vi "micIndividualTest.vi"() -> ()   [LabVIEW 2017]
uses:
  <vilib>/express/express analysis/Spectral/Block/exnSpectralBlock spectral measurements RMS poly.vi
  <vilib>/express/express analysis/Spectral/Block/exnSpectralBlock spectral measurements RMS DDT.vi
  <vilib>/express/express analysis/Spectral/XNode/ExpressSpectralMeasurementsBlockNode.xnode
panel:
  in  "Low pass filter":bool
  in  "Cut-Off Freq":dbl=800.0 caption="Lower Cut-Off"
  in  "Sampling Rate":dbl=25600.0
  in  "Tab Control":T1(tab)=enum."1-4"
  in  "Channel":u16(ring) items=["0", "1", "2", "3", "4", "5", "6", "7", "8", "9", "10", "11", "12", "13", "14", "15", "16"]
  out "Selected mic":dynamicdata(graph) caption="mic_4"
  out "fft selected mic":dynamicdata(graph)
  out "mic_3":dynamicdata(graph)
  out "fft_mic_3":dynamicdata(graph)
  out "fft_mic_4":dynamicdata(graph)
  out "mic_4":dynamicdata(graph)
  out "mic_1":dynamicdata(graph)
  out "fft_mic_1":dynamicdata(graph)
  out "fft_mic_2":dynamicdata(graph)
  out "mic_2":dynamicdata(graph)
  out "mic_6":dynamicdata(graph) caption="mic_2"
  out "fft_mic_6":dynamicdata(graph)
  out "fft_mic_5":dynamicdata(graph)
  out "mic_5":dynamicdata(graph) caption="mic_1"
  out "mic_8":dynamicdata(graph) caption="mic_4"
  out "fft_mic_8":dynamicdata(graph)
  out "fft_mic_7":dynamicdata(graph)
  out "mic_7":dynamicdata(graph) caption="mic_3"
  out "mic_11":dynamicdata(graph) caption="mic_3"
  out "fft_mic_11":dynamicdata(graph)
  out "fft_mic_12":dynamicdata(graph)
  out "mic_12":dynamicdata(graph) caption="mic_4"
  out "mic_9":dynamicdata(graph) caption="mic_1"
  out "fft_mic_9":dynamicdata(graph)
  out "fft_mic_10":dynamicdata(graph)
  out "mic_10":dynamicdata(graph) caption="mic_2"
  out "mic_14":dynamicdata(graph) caption="mic_2"
  out "fft_mic_14":dynamicdata(graph)
  out "fft_mic_13":dynamicdata(graph)
  out "mic_13":dynamicdata(graph) caption="mic_1"
  out "mic_16":dynamicdata(graph) caption="mic_4"
  out "fft_mic_16":dynamicdata(graph)
  out "fft_mic_15":dynamicdata(graph)
  out "mic_15":dynamicdata(graph) caption="mic_3"
  in  "stop (F)":bool caption="Stop (F)"
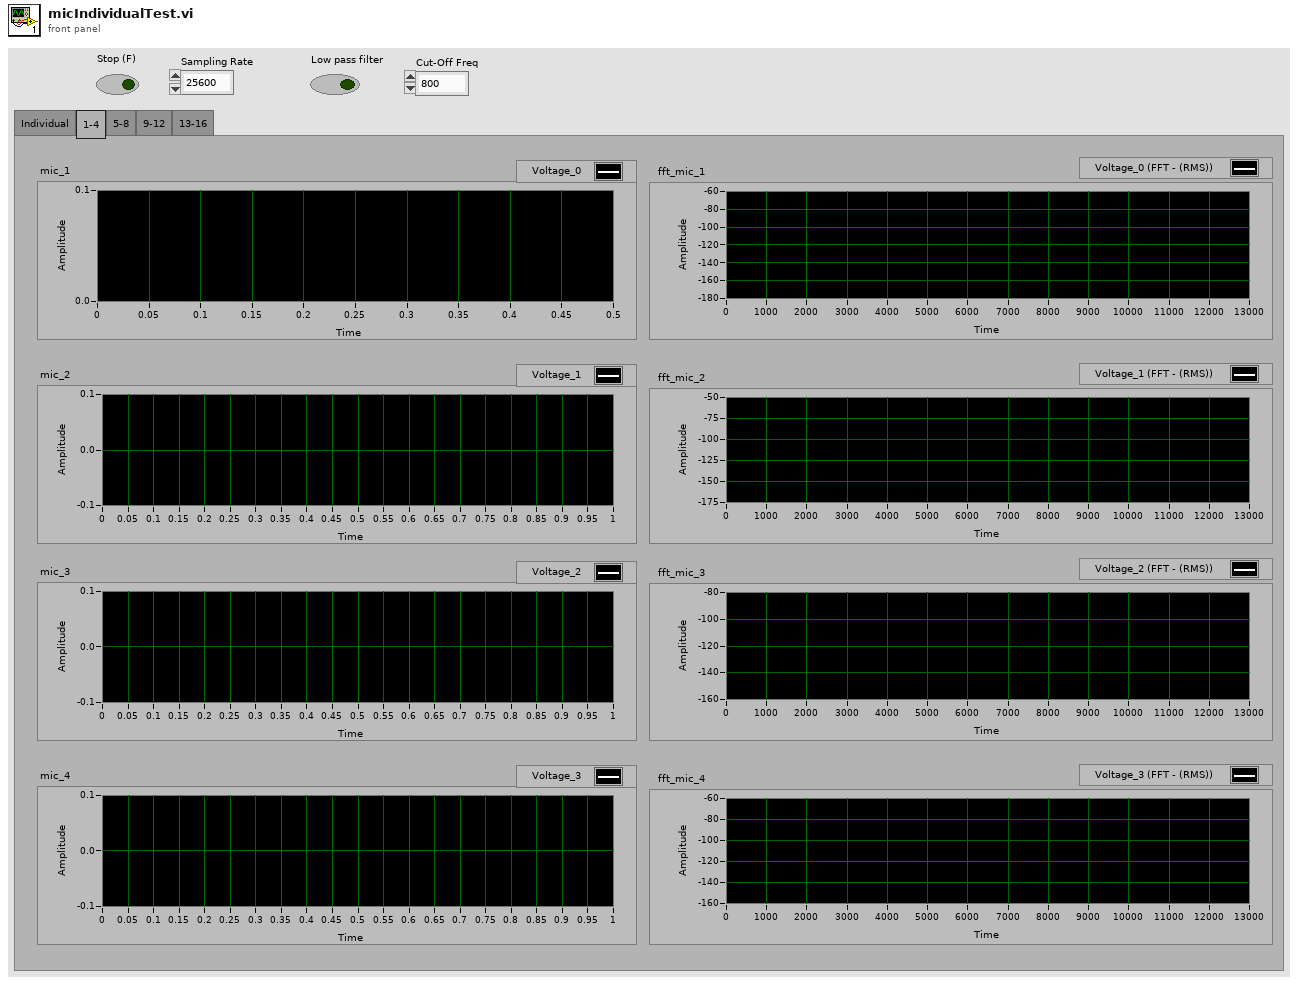
[diagram p1: front panel]
types:
  T1 = enum32{"Individual", "1-4", "5-8", "9-12", "13-16"}
  T2 = cluster{"averaging mode":u16, "weighting mode":u16, "number of averages":u32}
  T3 = cluster{"dB On (F)":bool, "unwrap phase (F)":bool, "convert to degree (F)":bool}
  T4 = enum8{"Enabled", "Disabled", "Disabled and Grayed Out"}
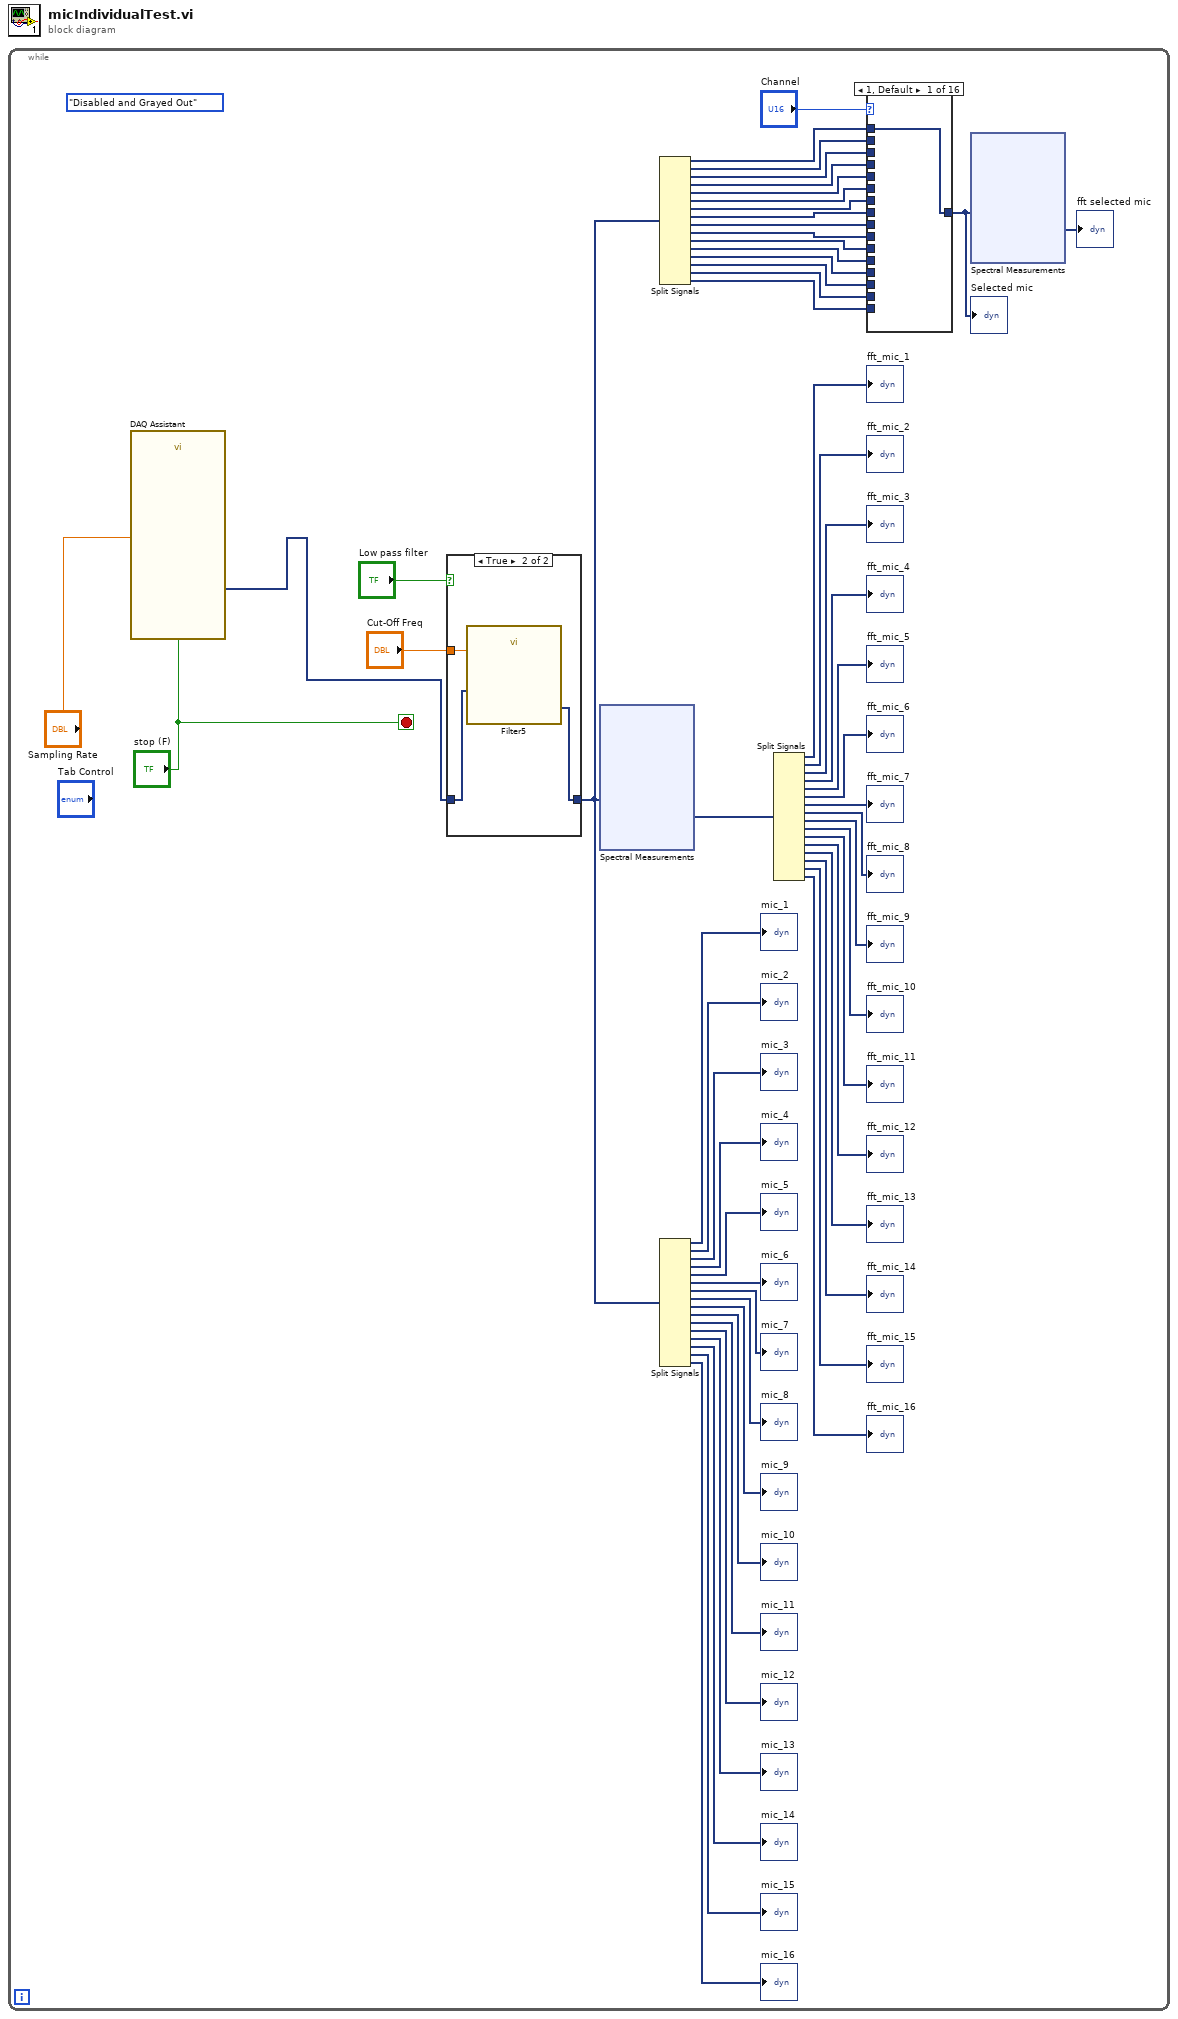
[diagram p0: block diagram]
diagram:
  n1 = while {
    stop <- "stop (F)" stop-if-true
    (unwired) T4."Disabled and Grayed Out" ("Disabled")
    n2 = call "DAQ Assistant"("rate"="Sampling Rate", "stop (T)"="stop (F)") -> ("data"=w3:dynamicdata)  [unwired: 15 in, 2 out]
    n3 = case shown="True" "Low pass filter" {
      tunnel: "Cut-Off Freq" -> [_ w88]
      tunnel: w3 -> [w85 w87]
      tunnel: [w85 w86] -> w5
      frame False {
      }
      frame True {
        n4 = call "Filter5"("Lower Cut-Off"=w88, "Signal"=w87) -> ("Filtered Signal"=w86:dynamicdata)  [unwired: 8 in, 1 out]
      }
    }
    n5 = xnode "Spectral Measurements"("Signals"=w5) -> ("FFT - (RMS)"=w24:dynamicdata)  [unwired: 1 in, 2 out]
    n6 = Split Signals(w5) -> (w23:dynamicdata, w22:dynamicdata, w21:dynamicdata, w20:dynamicdata, w19:dynamicdata, w18:dynamicdata, w17:dynamicdata, w16:dynamicdata, w15:dynamicdata, w14:dynamicdata, w13:dynamicdata, w12:dynamicdata, w11:dynamicdata, w10:dynamicdata, w9:dynamicdata, w8:dynamicdata)  [unwired: 16 in]
    n7 = Split Signals(w5) -> (→"mic_1":dynamicdata, →"mic_2":dynamicdata, →"mic_3":dynamicdata, →"mic_4":dynamicdata, →"mic_5":dynamicdata, →"mic_6":dynamicdata, →"mic_7":dynamicdata, →"mic_8":dynamicdata, →"mic_9":dynamicdata, →"mic_10":dynamicdata, →"mic_11":dynamicdata, →"mic_12":dynamicdata, →"mic_13":dynamicdata, →"mic_14":dynamicdata, →"mic_15":dynamicdata, →"mic_16":dynamicdata)  [unwired: 16 in]
    n8 = Split Signals(w24) -> (→"fft_mic_1":dynamicdata, →"fft_mic_2":dynamicdata, →"fft_mic_3":dynamicdata, →"fft_mic_4":dynamicdata, →"fft_mic_5":dynamicdata, →"fft_mic_6":dynamicdata, →"fft_mic_7":dynamicdata, →"fft_mic_8":dynamicdata, →"fft_mic_9":dynamicdata, →"fft_mic_10":dynamicdata, →"fft_mic_11":dynamicdata, →"fft_mic_12":dynamicdata, →"fft_mic_13":dynamicdata, →"fft_mic_14":dynamicdata, →"fft_mic_15":dynamicdata, →"fft_mic_16":dynamicdata)  [unwired: 16 in]
    n9 = case shown="1, Default" "Channel" {
      tunnel: w23 -> [w69 _ _ _ _ _ _ _ _ _ _ _ _ _ _ _]
      tunnel: w22 -> [_ w70 _ _ _ _ _ _ _ _ _ _ _ _ _ _]
      tunnel: w21 -> [_ _ w71 _ _ _ _ _ _ _ _ _ _ _ _ _]
      tunnel: w20 -> [_ _ _ w72 _ _ _ _ _ _ _ _ _ _ _ _]
      tunnel: w19 -> [_ _ _ _ w73 _ _ _ _ _ _ _ _ _ _ _]
      tunnel: w18 -> [_ _ _ _ _ w74 _ _ _ _ _ _ _ _ _ _]
      tunnel: w17 -> [_ _ _ _ _ _ w75 _ _ _ _ _ _ _ _ _]
      tunnel: w16 -> [_ _ _ _ _ _ _ w76 _ _ _ _ _ _ _ _]
      tunnel: w15 -> [_ _ _ _ _ _ _ _ w77 _ _ _ _ _ _ _]
      tunnel: w14 -> [_ _ _ _ _ _ _ _ _ w78 _ _ _ _ _ _]
      tunnel: w13 -> [_ _ _ _ _ _ _ _ _ _ w79 _ _ _ _ _]
      tunnel: w12 -> [_ _ _ _ _ _ _ _ _ _ _ w80 _ _ _ _]
      tunnel: w11 -> [_ _ _ _ _ _ _ _ _ _ _ _ w81 _ _ _]
      tunnel: w10 -> [_ _ _ _ _ _ _ _ _ _ _ _ _ w82 _ _]
      tunnel: w9 -> [_ _ _ _ _ _ _ _ _ _ _ _ _ _ w83 _]
      tunnel: w8 -> [_ _ _ _ _ _ _ _ _ _ _ _ _ _ _ w84]
      tunnel: [w69 w70 w71 w72 w73 w74 w75 w76 w77 w78 w79 w80 w81 w82 w83 w84] -> w6
      frame 1, Default {
      }
      frame 2 {
      }
      frame 3 {
      }
      frame 4 {
      }
      frame 5 {
      }
      frame 6 {
      }
      frame 7 {
      }
      frame 8 {
      }
      frame 9 {
      }
      frame 10 {
      }
      frame 11 {
      }
      frame 12 {
      }
      frame 13 {
      }
      frame 14 {
      }
      frame 15 {
      }
      frame 16 {
      }
    }
    "Selected mic" <- w6
    n10 = xnode "Spectral Measurements"("Signals"=w6) -> ("FFT - (RMS)"=→"fft selected mic":dynamicdata)  [unwired: 1 in, 2 out]
  }
